vi "validate key value pair.vi"(8 "error in":errorcluster, 9 "value":string, 10 "key":string, 11 "ThreePhasePLL configuration in":refnum<class "ThreePhasePLL configuration.lvclass">) -> (0 "error out":errorcluster, 3 "ThreePhasePLL configuration out":refnum<class "ThreePhasePLL configuration.lvclass">)   [LabVIEW 2017, in "ThreePhasePLL configuration.lvclass"]
uses:
  ThreePhasePLL configuration.lvclass
  <vilib>/NI/DCAF/Tag Editor Core/control module/configuration/control module configuration.lvclass
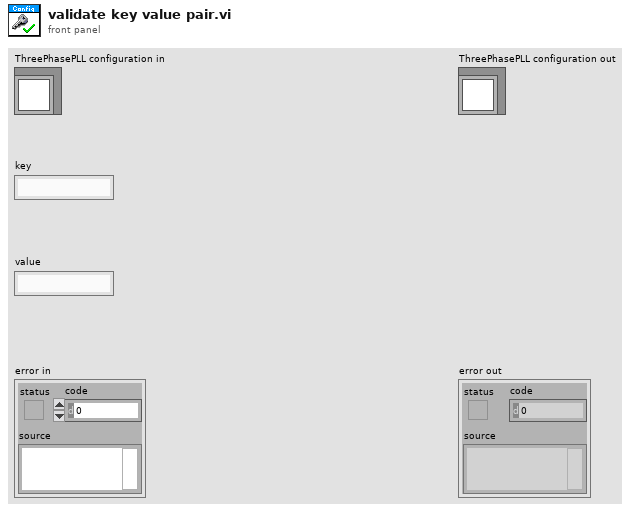
[diagram p1: front panel]
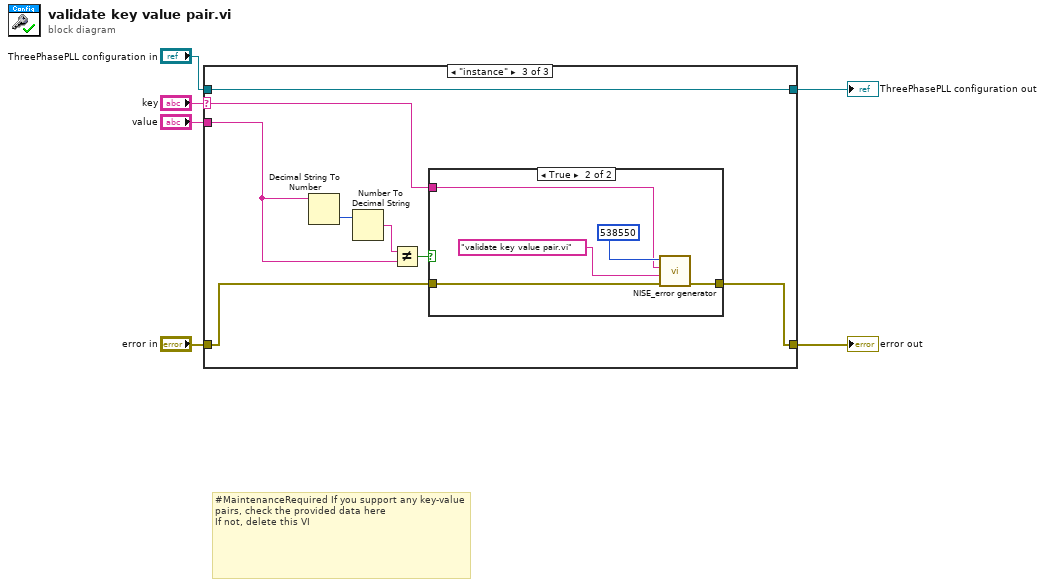
[diagram p0: block diagram]
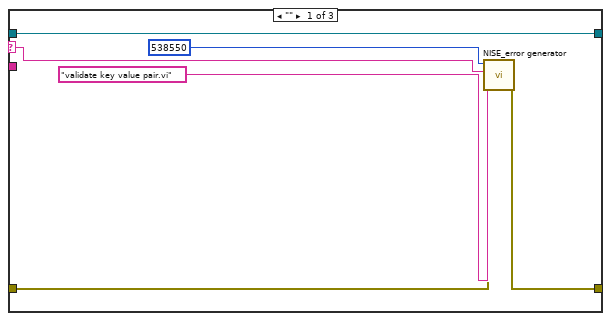
[diagram p2: hidden frame]
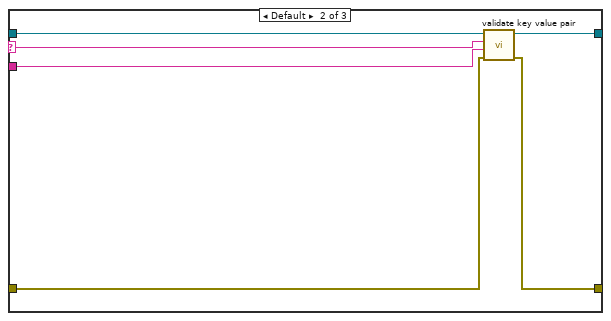
[diagram p3: hidden frame]
diagram:
  # "#MaintenanceRequired If you support any key-value pairs, check the provided data here\nIf not, delete this VI"
  n1 = case shown="\"instance\"" "key" {
    selector: "key" -> [w9 w13 w23]
    tunnel: [w7 w18 w20] -> w6
    tunnel: [w12 w17 w19] -> w5
    tunnel: "error in" -> [w8 w16 w21]
    tunnel: "value" -> [_ w15 w22]
    tunnel: "ThreePhasePLL configuration in" -> [w12 w14 w19]
    frame "" {
      n2 = call <vilib>:"NISE_error generator.vi"("error in"=w8, "source"="validate key value pair.vi", "append error message"=w9, "error code (0)"=538550) -> ("error out"=w7:errorcluster)  [unwired: 5 in]
    }
    frame Default {
      n3 = call-parent "validate key value pair.vi"("error in"=w16, "value"=w15, "key"=w13, "fixed channel configuration in"=w14) -> ("error out"=w18:errorcluster, "fixed channel configuration out"=w17:refnum<class "ThreePhasePLL configuration.lvclass">)  [unwired: 6 in]
    }
    frame "instance" {
      n4 = Decimal String To Number(string=w22) -> (number=w26:i32)  [unwired: 2 in, 1 out]
      n5 = Number To Decimal String(number=w26) -> (decimal integer string=w25:string)  [unwired: 1 in]
      n6 = Not Equal?(x=w25, y=w22) -> (x != y?=w24:bool)
      n7 = case shown="True" w24 {
        tunnel: w23 -> [_ w30]
        tunnel: [w27 w29] -> w20
        tunnel: w21 -> [w27 w28]
        frame False {
        }
        frame True {
          n8 = call <vilib>:"NISE_error generator.vi"("error in"=w28, "source"="validate key value pair.vi", "append error message"=w30, "error code (0)"=538550) -> ("error out"=w29:errorcluster)  [unwired: 5 in]
        }
      }
    }
  }
  "error out" <- w6
  "ThreePhasePLL configuration out" <- w5
